vi "MB Cull and Group.vi"(6 "min ratio":dbl=3.0 format="%#_13g", 7 "max ratio":dbl=8.0 format="%#_13g", 8 "Max":dbl=15.0, 9 "min":dbl=70.0, 10 "Sorted Data":dbl[][](array[numeric])) -> (2 "Best Targets above cutoff":T1(array[cluster]))   [LabVIEW 2017]
doc: "Examine the particle measurements to find the most likely pair that make up the target. This primarily compares the edges of the bounding boxes. It then returns information about the best two targets, notably the rectangle sourrounding the particles and the score."
panel:
  out "Array":dbl[](array[numeric])
  out "Grouping Scores":T2(array[cluster])
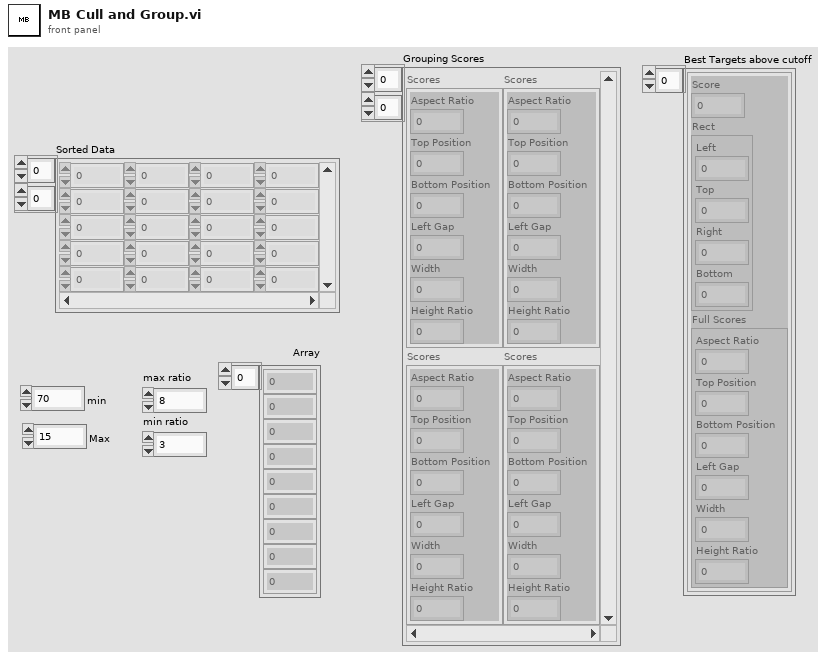
[diagram p1: front panel]
types:
  T1 = cluster{"Score":dbl, "Rect":cluster{"Left":dbl, "Top":dbl, "Right":dbl, "Bottom":dbl}, "Full Scores":cluster{"Aspect Ratio":dbl, "Top Position":dbl, "Bottom Position":dbl, "Left Gap":dbl, "Width":dbl, "Height Ratio":dbl}}[]
  T2 = cluster{"Aspect Ratio":dbl, "Top Position":dbl, "Bottom Position":dbl, "Left Gap":dbl, "Width":dbl, "Height Ratio":dbl}[][]
  T3 = typedef "Particle Parameters" = i32
  T4 = cluster{"Left":dbl, "Top":dbl, "Right":dbl, "Bottom":dbl}
  T5 = cluster{"f":dbl, "Rect":cluster{"Left":dbl, "Top":dbl, "Right":dbl, "Bottom":dbl}}
  T6 = cluster{"f":dbl, "Rect":cluster{"Left":dbl, "Top":dbl, "Right":dbl, "Bottom":dbl}}[]
  T7 = cluster{dbl, "Rect":cluster{"Left":dbl, "Top":dbl, "Right":dbl, "Bottom":dbl}, "Scores":cluster{"Aspect Ratio":dbl, "Strip Width":dbl, "Bottom Position":dbl, "Left Gap":dbl, "Width":dbl, "Height Ratio":dbl}}
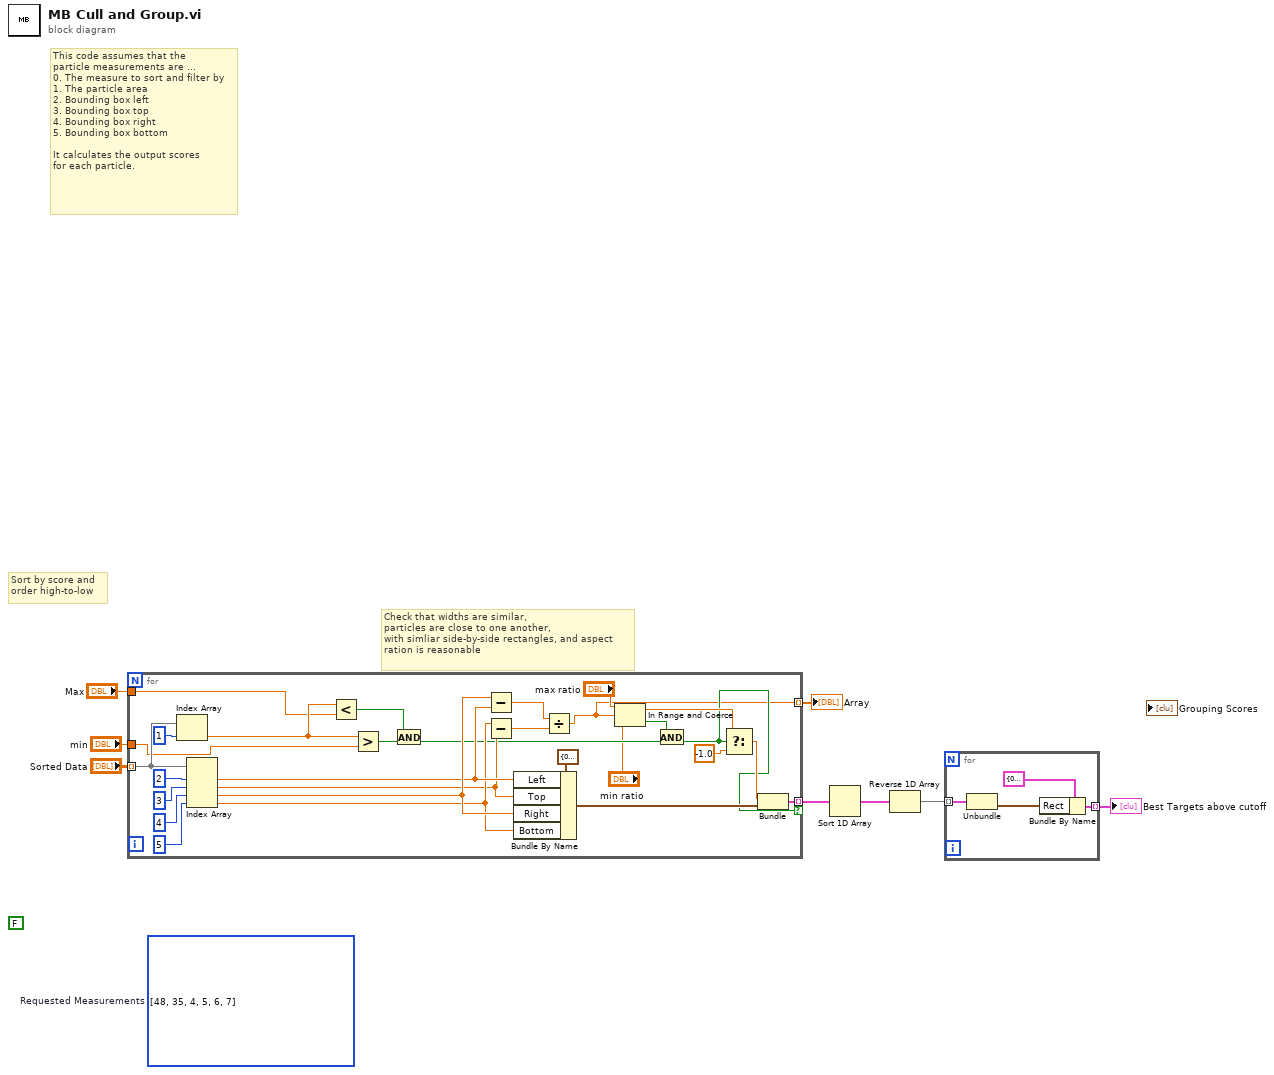
[diagram p0: block diagram]
diagram:
  (unwired) T3[] [48, 35, 4, 5, 6, 7] items=["Center of Mass X", "Center of Mass Y", "First Pixel X", "First Pixel Y", "Bounding Rect Left", "Bounding Rect Top", "Bounding Rect Right", "Bounding Rect Bottom", "Max Feret Diameter Start X", "Max Feret Diameter Start Y", "Max Feret Diameter End X", "Max Feret Diameter End Y", "Max Horiz. Segment Length Left", "Max Horiz. Segment Length Right", "Max Horiz. Segment Length Row", "-", "Bounding Rect Width", "Bounding Rect Height", "Bounding Rect Diagonal", "Perimeter", "Convex Hull Perimeter", "Holes' Perimeter", "Max Feret Diameter", "Equivalent Ellipse Major Axis", "Equivalent Ellipse Minor Axis", "Equivalent Ellipse Minor Axis (Feret)", "Equivalent Rect Long Side", "Equivalent Rect Short Side", "Equivalent Rect Diagonal", "Equivalent Rect Short Side (Feret)", "Average Horiz. Segment Length", "Average Vert. Segment Length", "Hydraulic Radius", "Waddel Disk Diameter", "-", "Area", "Holes' Area", "Particle & Holes' Area", "Convex Hull Area", "Image Area", "-", "Number of Holes", "Number of Horiz. Segments", "Number of Vert. Segments", "-", "Orientation", "Max Feret Diameter Orientation", "-", "% Area/Image Area", "% Area/(Particle & Holes' Area)", "Ratio of Equivalent Ellipse Axes", "Ratio of Equivalent Rect Sides", "-", "Elongation Factor", "Compactness Factor", "Heywood Circularity Factor", "Type Factor", "-", "Sum X", "Sum Y", "Sum XX", "Sum XY", "Sum YY", "Sum XXX", "Sum XXY", "Sum XYY", "Sum YYY", "-", "Moment of Inertia XX", "Moment of Inertia XY", "Moment of Inertia YY", "Moment of Inertia XXX", "Moment of Inertia XXY", "Moment of Inertia XYY", "Moment of Inertia YYY", "Norm. Moment of Inertia XX", "Norm. Moment of Inertia XY", "Norm. Moment of Inertia YY", "Norm. Moment of Inertia XXX", "Norm. Moment of Inertia XXY", "Norm. Moment of Inertia XYY", "Norm. Moment of Inertia YYY", "Hu Moment 1", "Hu Moment 2", "Hu Moment 3", "Hu Moment 4", "Hu Moment 5", "Hu Moment 6", "Hu Moment 7"]  # Requested Measurements
  (unwired) FALSE
  # "Sort by score and\norder high-to-low"
  # "Check that widths are similar,\nparticles are close to one another,\nwith simliar side-by-side rectangles, and aspect\nration is reasonable"
  # "This code assumes that the\nparticle measurements are ...\n0. The measure to sort and filter by\n1. The particle area\n2. Bounding box left\n3. Bounding box top\n4. Bounding box right\n5. Bounding box bottom\n\nIt calculates the output scores\nfor each particle."
  n1 = for {
    tunnel: "Sorted Data" -> [w24] mode=indexing
    tunnel: [w25] -> w7 mode=indexing if=w11
    tunnel: "min" -> [w22]
    tunnel: "Max" -> [w15]
    tunnel: [w9] -> w1 mode=indexing
    n2 = Index Array(array=w24, index=1) -> (element=w16:dbl)
    n3 = Index Array(array=w24, index #1=2 ("index"), index #2=3 ("index"), index #3=4 ("index"), index #4=5 ("index")) -> (element #1=w31:dbl, element #2=w29:dbl, element #3=w32:dbl, element #4=w30:dbl)
    n4 = Less?(x=w16, y=w15) -> (x < y?=w17:bool)
    n5 = Greater?(x=w16, y=w22) -> (0:w19:bool)
    n6 = And(x=w17, y=w19) -> (x .and. y?=w18:bool)
    n7 = Subtract(x=w32, y=w31) -> (x-y=w28:dbl)
    n8 = Subtract(x=w30, y=w29) -> (x-y=w27:dbl)
    n9 = Bundle By Name(cluster=T4 {"Left"=0.0, "Top"=0.0, "Right"=0.0, "Bottom"=0.0} ("Rect"), "Left"=w31, "Top"=w29, "Right"=w32, "Bottom"=w30) -> (w26:T4)
    n10 = Divide(x=w28, y=w27) -> (x/y=w9:dbl)
    n11 = In Range and Coerce(upper limit="max ratio", x=w9, lower limit="min ratio") -> (coerced(x)=w14:dbl, In Range?=w10:bool)
    n12 = And(x=w10, y=w18) -> (x .and. y?=w11:bool)
    n13 = Select(t=w14, s=w11, f=-1.0) -> (s? t:f=w20:dbl)
    n14 = Bundle("f"=w20, "Rect"=w26) -> (w25:T5)  [unwired: 1 in]
  }
  "Array" <- w1
  n15 = Sort 1D Array(array=w7) -> (sorted array=w6:T6)
  n16 = Reverse 1D Array(array=w6) -> (reversed array=w2:T6)
  n17 = for {
    tunnel: w2 -> [w41] mode=indexing
    tunnel: [w38] -> w5 mode=indexing
    n18 = Unbundle(w41) -> ("Rect"=w39:T4)  [unwired: 1 out]
    n19 = Bundle By Name(cluster=T7 {0.0, "Rect"={"Left"=0.0, "Top"=0.0, "Right"=0.0, "Bottom"=0.0}, "Scores"={"Aspect Ratio"=0.0, "Strip Width"=0.0, "Bottom Position"=0.0, "Left Gap"=0.0, "Width"=0.0, "Height Ratio"=0.0}}, "Rect"=w39) -> (w38:T7)
  }
  "Best Targets above cutoff" <- w5
